vi "Create Tree Manager.vi"(8 "error in (no error)":errorcluster, 11 "Tree Control":refnum<vi>) -> (0 "error out":errorcluster, 3 "Tree Manager":refnum<class "Tree Manager.lvclass">)   [LabVIEW 2026, in "VILab.lvlib" / "Tree Manager.lvclass"]
uses:
  Tree Manager.lvclass
  Tree Manager.lvclass/Tree Manager.ctl
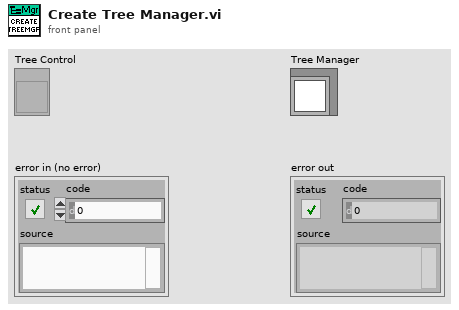
[diagram p1: front panel]
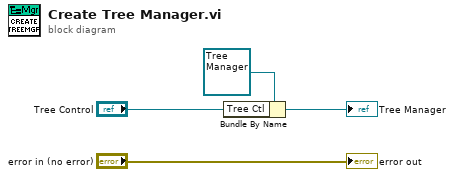
[diagram p0: block diagram]
diagram:
  n1 = Bundle By Name(cluster=refnum<class "Tree Manager.lvclass"> refnum ("VILab.lvlib:Tree Manager.lvclass"), "Tree Ctl"="Tree Control") -> (→"Tree Manager":refnum<class "Tree Manager.lvclass">)
  "error out" <- "error in (no error)"
